vi "Load Digital Project.vi"(0 "instrument handle":refnum<k15>, 11 "error in":errorcluster) -> (4 "instrument handle out":refnum<k15>, 15 "error out":errorcluster)   [LabVIEW 2018, in "MIPI RFFE API.lvlib"]
uses:
  MIPI RFFE API.lvlib
  <instrlib>/niDigital/niDigital.llb/niDigital Load Specifications Levels and Timing (Single).vi
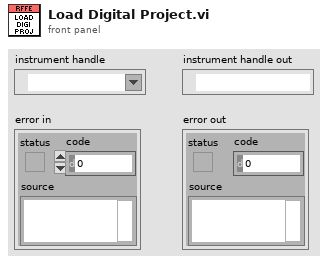
[diagram p1: front panel]
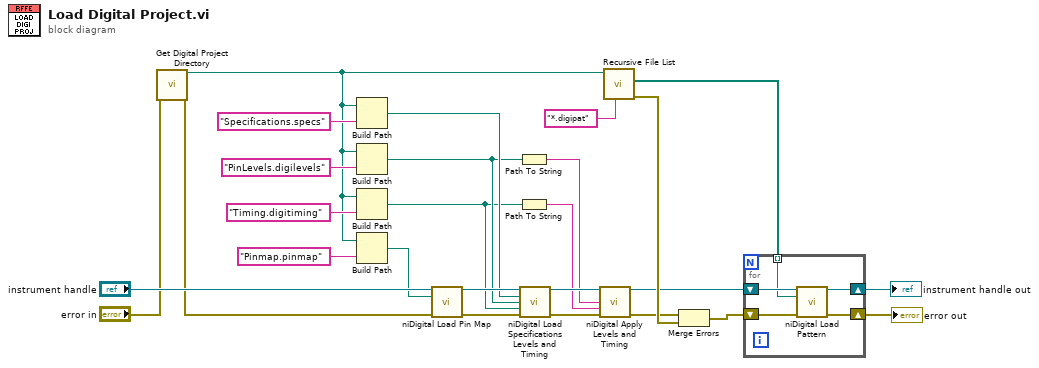
[diagram p0: block diagram]
diagram:
  n1 = call "Get Digital Project Directory.vi"("error in (no error)"="error in") -> ("Digital Project Directory"=w2:path, "error out"=w1:errorcluster)  [unwired: 13 in]
  n2 = Build Path(base path=w2, name or relative path="Specifications.specs") -> (appended path=w17:path)
  n3 = Build Path(base path=w2, name or relative path="PinLevels.digilevels") -> (appended path=w6:path)
  n4 = Build Path(base path=w2, name or relative path="Timing.digitiming") -> (appended path=w5:path)
  n5 = Build Path(base path=w2, name or relative path="Pinmap.pinmap") -> (appended path=w19:path)
  n6 = call <instrlib>:"niDigital Load Pin Map.vi"("instrument handle"="instrument handle", "pin map file"=w19, "error in"=w1) -> ("instrument handle out"=w22:refnum<k15>, "error out"=w21:errorcluster)  [unwired: 11 in]
  n7 = Path To String(path=w6) -> (string=w4:string)
  n8 = Path To String(path=w5) -> (string=w3:string)
  n9 = call-poly <instrlib>:"niDigital Load Specifications Levels and Timing.vi"("instrument handle"=w22, "specifications file path"=w17, "levels file path"=w6, "timing file path"=w5, "error in"=w21) -> ("instrument handle out"=w8:refnum<k15>, "error out"=w12:errorcluster)  [unwired: 9 in]
  n10 = call <instrlib>:"niDigital Apply Levels and Timing.vi"("instrument handle"=w8, "levels sheet"=w4, "timing sheet"=w3, "error in"=w12) -> ("instrument handle out"=w7:refnum<k15>, "error out"=w9:errorcluster)  [unwired: 10 in]
  n11 = call <vilib>:"Recursive File List.vi"("pattern"="*.digipat", "Folder Path"=w2) -> ("error out"=w11:errorcluster, "All Files in Dir"=w13:path[])  [unwired: 5 in, 3 out]
  n12 = Merge Errors(w9, w11) -> (w10:errorcluster)
  n13 = for {
    shift-right: [w29] -> w24
    shift-left: w7 -> [w31]
    shift-right: [w28] -> w23
    shift-left: w10 -> [w30]
    tunnel: w13 -> [w27] mode=indexing
    n14 = call <instrlib>:"niDigital Load Pattern.vi"("instrument handle"=w31, "pattern file"=w27, "error in"=w30) -> ("instrument handle out"=w29:refnum<k15>, "error out"=w28:errorcluster)  [unwired: 11 in]
  }
  "instrument handle out" <- w24
  "error out" <- w23
